vi "degrees_to_hex_encoder.vi"(8 "Encoder Pulses per Degree":i32=398, 11 "Degrees":dbl) -> (0 "Encoded Degrees":dbl, 3 "hex integer string":string)   [LabVIEW 2024]
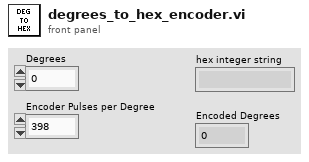
[diagram p1: front panel]
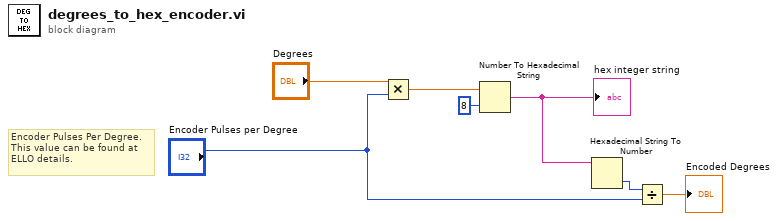
[diagram p0: block diagram]
diagram:
  # "Encoder Pulses Per Degree.\nThis value can be found at\nELLO details."
  n1 = Multiply(x="Degrees", y="Encoder Pulses per Degree") -> (x*y=w6:dbl)
  n2 = Number To Hexadecimal String(1:i16 8 ("width (-)"), 2:w6) -> (0:w5:string)
  "hex integer string" <- w5
  n3 = Hexadecimal String To Number(string=w5) -> (number=w4:u32)  [unwired: 2 in, 1 out]
  n4 = Divide(x=w4, y="Encoder Pulses per Degree") -> (x/y=→"Encoded Degrees":dbl)
